vi "Calculate Receiver Calibration Coefficients.vi"(7 "Channel (1)":i32=1, 8 "error in (no error)":errorcluster, 9 "Port 1 (1)":i32=1, 10 "Receiver (1)":i32=1, 11 "VISA resource name":refnum<visa-resource-name>) -> (0 "error out":errorcluster, 3 "VISA resource name out":refnum<visa-resource-name>)   [LabVIEW 2022 SP3, in "Agilent ENA Series.lvlib"]
doc: "Calculates the receiver calibration error, for selected channel,\ncoefficient for the specified port (executes receiver calibration).\n\nThe measurement port and the source port are THRU-connected for execution. Therefore, if the same port number is specified for the measurement port and the source port, an error occurs.\n\nBecause information of power calibration for both the measurement port and the source port is used for error coefficient calculation, the precision of receiver calibration is improved by executing power calibration for the both ports before executing receiver calibration.\n\n<b>Note:</b>\nThis VI is not supported by the E5063A model."
uses:
  <instrlib>/Agilent ENA Series/Agilent ENA Series.lvlib
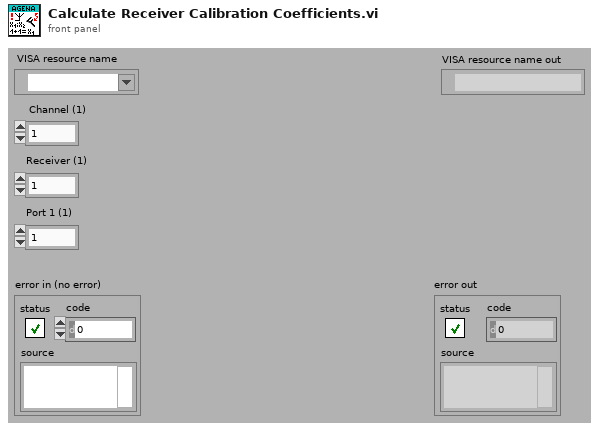
[diagram p1: front panel]
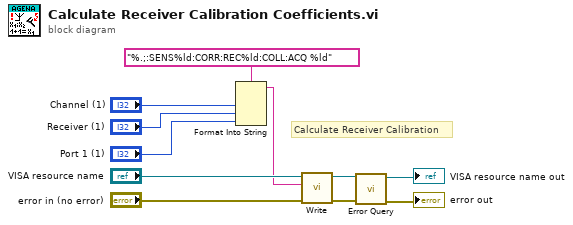
[diagram p0: block diagram]
diagram:
  # "Calculate Receiver Calibration"
  n1 = Format Into String(format string="%.;:SENS%ld:CORR:REC%ld:COLL:ACQ %ld", "Channel (1)", "Receiver (1)", "Port 1 (1)") -> (resulting string=w7:string)  [unwired: 2 in, 1 out]
  n2 = call <instrlib>:"Write.vi"("error in (no error)"="error in (no error)", "String ()"=w7, "VISA resource name"="VISA resource name") -> ("error out"=w3:errorcluster, "VISA resource name out"=w4:refnum<visa-resource-name>)  [unwired: 6 in, 1 out]
  n3 = call <instrlib>:"Error Query.vi"("error in (no error)"=w3, "VISA resource name"=w4) -> ("error out"=→"error out":errorcluster, "VISA resource name out"=→"VISA resource name out":refnum<visa-resource-name>)  [unwired: 6 in, 2 out]
